vi "Shutdown Module.vi"(8 "error in (no error)":errorcluster, 9 "params":variant, 11 "Controller in":refnum<class "Controller.lvclass">) -> (0 "error out":errorcluster, 3 "Controller out":refnum<class "Controller.lvclass">)   [LabVIEW 2020, in "Controller.lvlib" / "Controller.lvclass"]
uses:
  Controller.lvclass
  Controller.lvclass/Controller.ctl
  RPC/TypeDefs/Request.ctl
  RPC.lvlib
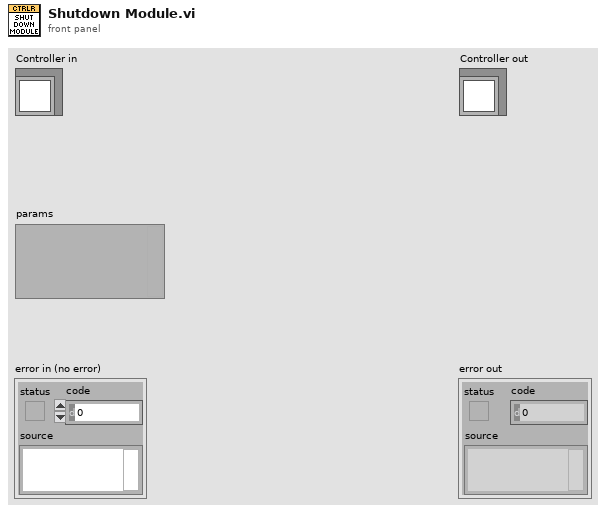
[diagram p1: front panel]
types:
  T1 = typedef "RPC.lvlib/Request.ctl" = cluster{"Method":string, "Params":variant}
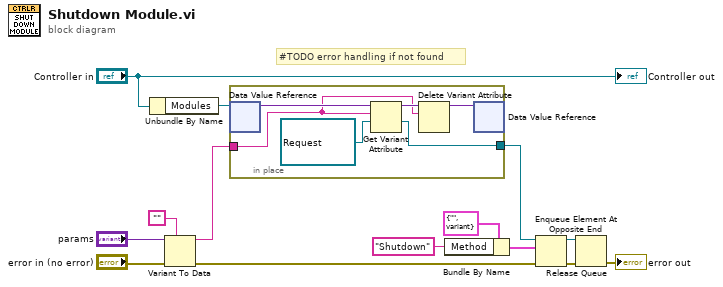
[diagram p0: block diagram]
diagram:
  # "#TODO error handling if not found"
  n1 = Unbundle By Name("Controller in") -> ("Modules"=w13:refnum<data-value>)
  n2 = Variant To Data(error in="error in (no error)", type="", Variant="params") -> (data=w10:string, error out=w3:errorcluster)
  n3 = in-place {
    in-place-border: w10 -> [w17]
    in-place-border: [w15] -> w4
    n4 = in-place-dvr #1(w13) -> (w19:variant)  [unwired: 1 out]
    n5 = Get Variant Attribute(Variant=w19, name=w17, default value (empty Variant)=refnum<queue> refnum ("queue out")) -> (duplicate Variant=w18:variant, value=w15:refnum<queue>)  [unwired: 1 in, 2 out]
    n6 = Delete Variant Attribute(6:w17, 7:w18) -> (3:w20:variant)  [unwired: 1 in, 2 out]
    n7 = in-place-dvr #1(w20) -> ()  [unwired: 2 out]
  }
  n8 = Bundle By Name(cluster=T1 {"Method"="", "Params"=variant} ("element"), "Method"="Shutdown" ("Message")) -> (w9:T1)
  n9 = Enqueue Element At Opposite End(queue=w4, element=w9, error in (no error)=w3) -> (queue out=w5:refnum<queue>, error out=w6:errorcluster)  [unwired: 1 in, 1 out]
  n10 = Release Queue(queue=w5, error in (no error)=w6) -> (error out=→"error out":errorcluster)  [unwired: 1 in, 2 out]
  "Controller out" <- "Controller in"
